vi "Run.vi"(0 "reg in":refnum<class "bronkhorst_reg_2.lvclass">, 1 "XB24 (F)":bool, 5 "ZY_control":T5={"Start"=FALSE, "Z_HSw"=0, "Z_HSetState"=enum."on", "Y_HSw"=0, "Y_HSetState"=enum."hand", "SP"=0.0, "Y_H"=0.0, "Reset_ALR"=FALSE} {"Y_H" step=1.0; "SP" step=0.01 format="%.2f"}, 7 "Y_in":dbl step=0.01 format="%.2f", 9 "Y_State":T4) -> (4 "reg out":refnum<class "bronkhorst_reg_2.lvclass">, 6 "Y":T1={"Y_Source"=enum."hand", "Y_SetState"=enum."hand", "SP_Set"=0.0, "SP"=0.0, "PV"=0.0, "PV_State"={"code"=0, "visible"=FALSE, "color"=0}, "Y_preSet"=0.0, "Y_Set"=0.0, "Y"=0.0, "Y_State"={"code"=0, "visible"=FALSE, "color"=0}, "YB"=FALSE} {"Y" format="%.2f"; "Y_preSet" format="%.2f"; "SP" step=0.01 format="%.2f"; "Y_Set" format="%.2f"; "PV" step=0.01 format="%.2f"; "SP_Set" step=0.01 format="%.2f"}, 8 "Y_out":dbl format="%.2f")   [LabVIEW 2019, in "control.lvlib" / "bronkhorst_reg_2.lvclass"]
uses:
  bronkhorst_reg_2.lvclass
  Inputs/Ctl/Parameter State short.ctl
  ctl/Y_Lim_State.ctl
  D:/my_projects/projects/Algorithms/Labview/19/Reg/Y_Limiter/Y_Limiter.lvclass
  ctl/ZY_control_short.ctl
  ctl/Z_State.ctl
  ctl/Y_state.ctl
  ctl/Y.ctl
  ctl/Y_source.ctl
  Y_Limiter/Y_Limiter.lvclass/Y_Limiter.ctl
  bronkhorst_reg_2.lvclass/bronkhorst_reg_2.ctl
  ctl/Y_control.ctl
  Inputs/Ctl/Sensor state.ctl
  Inputs/Ctl/Sensor alarm.ctl
  PID/PID Output Rate Limiter/PID Output Rate Limiter.lvclass/PID Output Rate Limiter.ctl
  PID/PID Timing Estimation/PID Timing Estimation.lvclass/PID Timing Estimation.ctl
  PID/PID Output Rate Limiter/PID Output Rate Limiter.vi
  PID/PID Output Rate Limiter/Read output.vi
  PID/PID Output Rate Limiter/Write output rate.vi
  PID/PID Output Rate Limiter/Read output rate.vi
  PID/PID Timing Estimation/PID Timing Estimation.vi
  Y_Limiter/Y_Limiter.lvclass
  D:/my_projects/projects/Algorithms/Labview/19/Reg/PID/PID Output Rate Limiter/PID Output Rate Limiter.lvclass
  PID/PID Output Rate Limiter/PID Output Rate Limiter.lvclass
  D:/my_projects/projects/Algorithms/Labview/19/Reg/PID/PID Timing Estimation/PID Timing Estimation.lvclass
  control.lvlib
  Inputs/Inputs.lvlib
panel:
  out "YLim_State":T7=enum."increase"
  out "End":bool
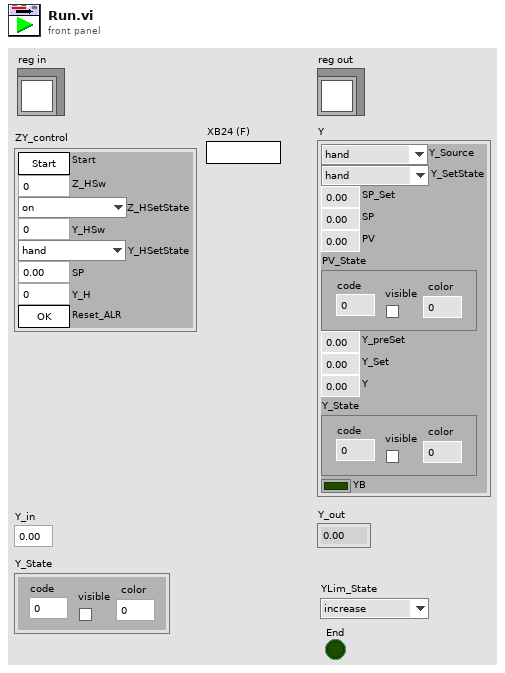
[diagram p1: front panel]
types:
  T1 = typedef "control.lvlib/Y.ctl" = cluster{"Y_Source":T2, "Y_SetState":T3, "SP_Set":dbl, "SP":dbl, "PV":dbl, "PV_State":T4, "Y_preSet":dbl, "Y_Set":dbl, "Y":dbl, "Y_State":T4, "YB":bool}
  T2 = typedef "control.lvlib/Y_source.ctl" = enum8{"initialize", "local disabled", "local hand", "hand", "auto", "dist"}
  T3 = typedef "control.lvlib/Y_state.ctl" = enum8{"initialize", "alarm", "min", "stop", "hand", "auto", "max"}
  T4 = typedef "Inputs.lvlib/Parameter State short.ctl" = cluster{"code":i32, "visible":bool, "color":u32}
  T5 = typedef "control.lvlib/ZY_control_short.ctl" = cluster{"Start":bool, "Z_HSw":u32, "Z_HSetState":T6, "Y_HSw":u32, "Y_HSetState":T3, "SP":dbl, "Y_H":dbl, "Reset_ALR":bool}
  T6 = typedef "control.lvlib/Z_State.ctl" = enum8{"initialization", "alarm", "disabled", "not ready", "stop ready", "reserv", "switched off", "reserv2", "switched on", "check", "on min", "decrease out", "on", "increase out", "on max"}
  T7 = typedef "control.lvlib/Y_Lim_State.ctl" = enum8{"initialization", "alarm", "stop", "decrease", "increase"}
  T8 = typedef "control.lvlib/Y_control.ctl" = cluster{"Y_HSw":u32, "Y_HSetState":T3, "Y_ASetState":T3, "Y_DSetState":T3}
  T9 = typedef "Inputs.lvlib/Sensor state.ctl" = cluster{"source":string, "color":u32, "visible":bool}[]
  T10 = typedef "Inputs.lvlib/Sensor alarm.ctl" = cluster{"source":string, "color":u32, "visible":bool}[]
  T11 = enum8{"alarm", "min", "stop", "hand", "auto", "max"}
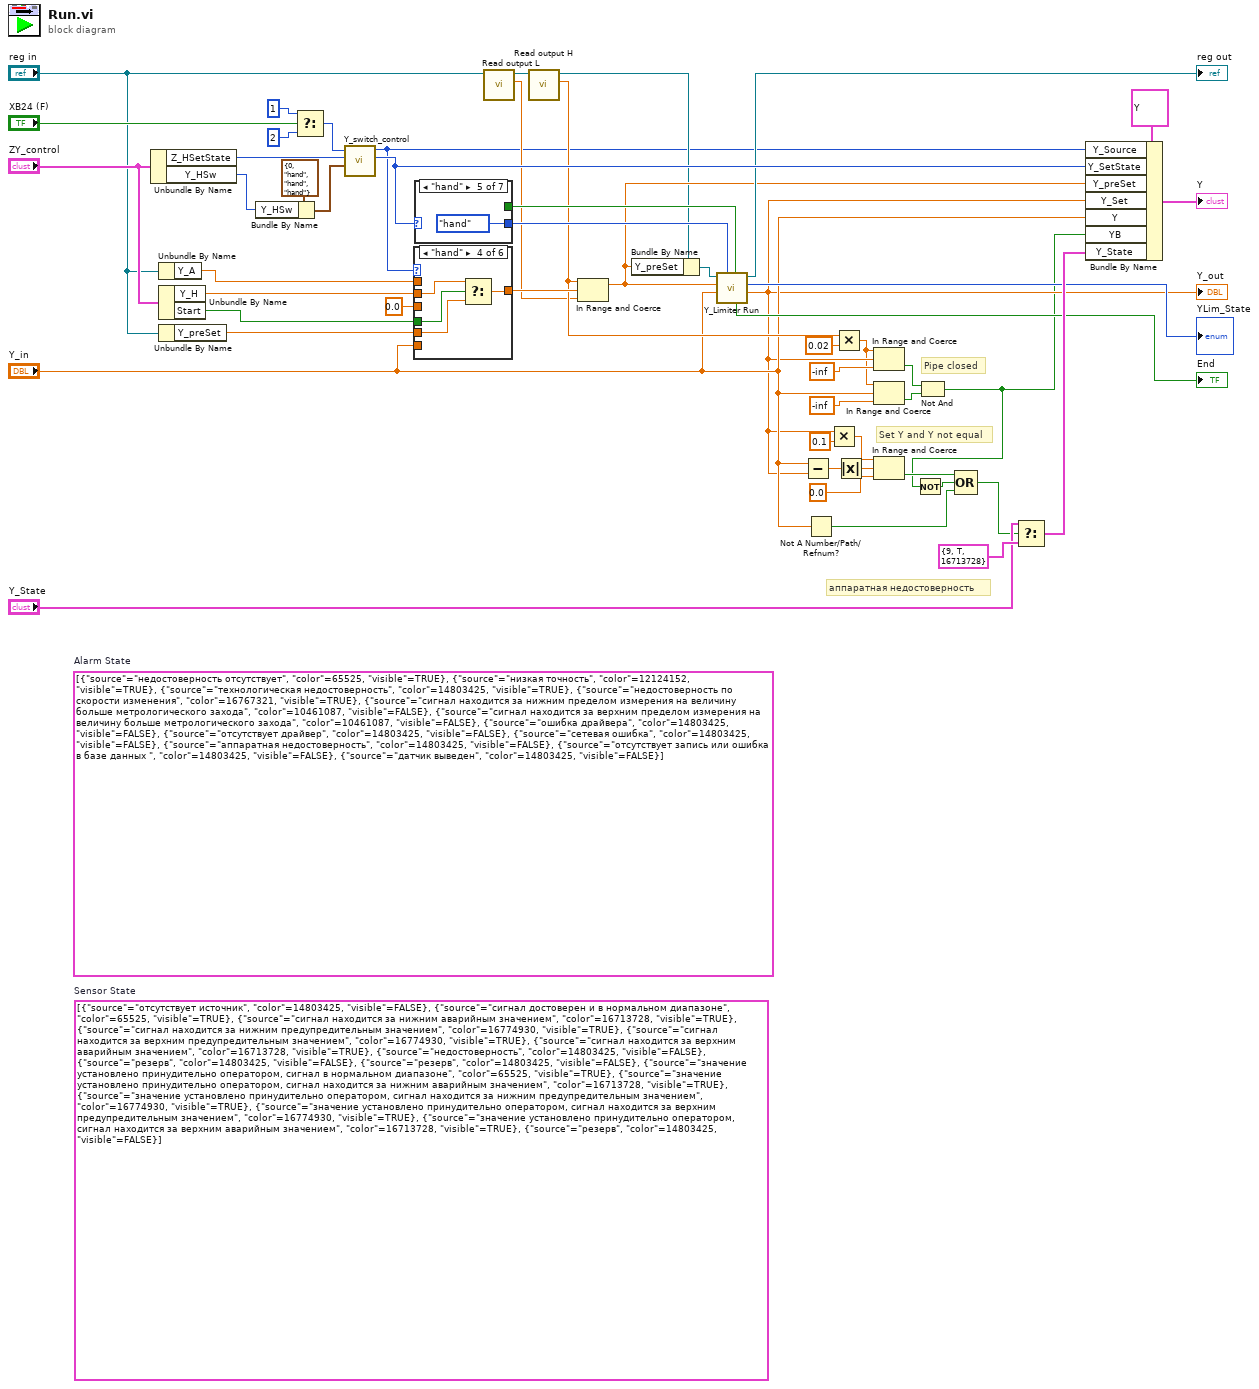
[diagram p0: block diagram]
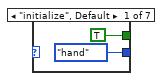
[diagram p2: hidden frame]
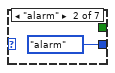
[diagram p3: hidden frame]
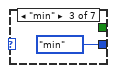
[diagram p4: hidden frame]
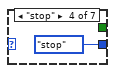
[diagram p5: hidden frame]
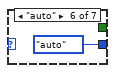
[diagram p6: hidden frame]
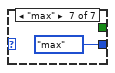
[diagram p7: hidden frame]
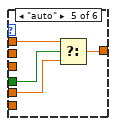
[diagram p11: hidden frame]
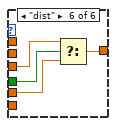
[diagram p12: hidden frame]
diagram:
  (unwired) T9 [{"source"="отсутствует источник", "color"=14803425, "visible"=FALSE}, {"source"="сигнал достоверен и в нормальном диапазоне", "color"=65525, "visible"=TRUE}, {"source"="сигнал находится за нижним аварийным значением", "color"=16713728, "visible"=TRUE}, {"source"="сигнал находится за нижним предупредительным значением", "color"=16774930, "visible"=TRUE}, {"source"="сигнал находится за верхним предупредительным значением", "color"=16774930, "visible"=TRUE}, {"source"="сигнал находится за верхним аварийным значением", "color"=16713728, "visible"=TRUE}, {"source"="недостоверность", "color"=14803425, "visible"=FALSE}, {"source"="резерв", "color"=14803425, "visible"=FALSE}, {"source"="резерв", "color"=14803425, "visible"=FALSE}, {"source"="значение установлено принудительно оператором, сигнал в нормальном диапазоне", "color"=65525, "visible"=TRUE}, {"source"="значение установлено принудительно оператором, сигнал находится за нижним аварийным значением", "color"=16713728, "visible"=TRUE}, {"source"="значение установлено принудительно оператором, сигнал находится за нижним предупредительным значением", "color"=16774930, "visible"=TRUE}, {"source"="значение установлено принудительно оператором, сигнал находится за верхним предупредительным значением", "color"=16774930, "visible"=TRUE}, {"source"="значение установлено принудительно оператором, сигнал находится за верхним аварийным значением", "color"=16713728, "visible"=TRUE}, {"source"="резерв", "color"=14803425, "visible"=FALSE}]  # Sensor State
  (unwired) T10 [{"source"="недостоверность отсутствует", "color"=65525, "visible"=TRUE}, {"source"="низкая точность", "color"=12124152, "visible"=TRUE}, {"source"="технологическая недостоверность", "color"=14803425, "visible"=TRUE}, {"source"="недостоверность по скорости изменения", "color"=16767321, "visible"=TRUE}, {"source"="сигнал находится за нижним пределом измерения на величину больше метрологического захода", "color"=10461087, "visible"=FALSE}, {"source"="сигнал находится за верхним пределом измерения на величину больше метрологического захода", "color"=10461087, "visible"=FALSE}, {"source"="ошибка драйвера", "color"=14803425, "visible"=FALSE}, {"source"="отсутствует драйвер", "color"=14803425, "visible"=FALSE}, {"source"="сетевая ошибка", "color"=14803425, "visible"=FALSE}, {"source"="аппаратная недостоверность", "color"=14803425, "visible"=FALSE}, {"source"="отсутствует запись или ошибка в базе данных ", "color"=14803425, "visible"=FALSE}, {"source"="датчик выведен", "color"=14803425, "visible"=FALSE}]  # Alarm State
  # "аппаратная недостоверность"
  # "Set Y and Y not equal"
  # "Pipe closed"
  n1 = Unbundle By Name("ZY_control") -> ("Z_HSetState"=w46:T6, "Y_HSw"=w47:u32)
  n2 = Unbundle By Name("reg in") -> ("Y_A"=w20:dbl)
  n3 = Unbundle By Name("ZY_control") -> ("Y_H"=w42:dbl, "Start"=w43:bool)
  n4 = Unbundle By Name("reg in") -> ("Y_preSet"=w21:dbl)
  n5 = Bundle By Name(cluster=T8 {"Y_HSw"=0, "Y_HSetState"=enum."hand", "Y_ASetState"=enum."hand", "Y_DSetState"=enum."hand"} ("Y"), "Y_HSw"=w47) -> (w45:T8)
  n6 = Select(t=u32 1, s="XB24 (F)", f=u32 2 ("Y_HSw")) -> (s? t:f=w50:u32)
  n7 = call "Y_switch_control.vi"("Y"=w45, "Z_State"=w46, "Y_LSw (2-auto)"=w50) -> ("Y_SetState"=w48:T3, "Y_Source"=w12:T2)  [unwired: 7 in]
  n8 = case shown="\"hand\"" w12 {
    tunnel: w42 -> [_ _ _ w56 _ _]
    tunnel: "Y_in" -> [w53 w54 w55 _ _ _]
    tunnel: 0.0 ("Y_A") -> [_ _ _ _ _ w66]
    tunnel: [w53 w54 w55 w59 w63 w67] -> w22
    tunnel: w20 -> [_ _ _ _ w60 _]
    tunnel: w21 -> [_ _ _ w58 w62 w65]
    tunnel: w43 -> [_ _ _ w57 w61 w64]
    frame "initialize", Default {
    }
    frame "local disabled" {
    }
    frame "local hand" {
    }
    frame "hand" {
      n9 = Select(t=w56, s=w57, f=w58) -> (s? t:f=w59:dbl)
    }
    frame "auto" {
      n10 = Select(t=w60, s=w61, f=w62) -> (s? t:f=w63:dbl)
    }
    frame "dist" {
      n11 = Select(t=w66, s=w64, f=w65) -> (s? t:f=w67:dbl)
    }
  }
  n12 = case shown="\"hand\"" w48 {
    tunnel: [T11."hand" ("X1(SetState)") T11."alarm" ("X1(SetState)") T11."min" ("X1(SetState)") T11."stop" ("X1(SetState)") T11."hand" ("X1(SetState)") T11."auto" ("X1(SetState)") T11."max" ("X1(SetState)")] -> w29
    tunnel: [TRUE _ _ _ _ _ _] -> w28
    frame "initialize", Default {
    }
    frame "alarm" {
    }
    frame "min" {
    }
    frame "stop" {
    }
    frame "hand" {
    }
    frame "auto" {
    }
    frame "max" {
    }
  }
  n13 = call "Read output L.vi"("Y_Limiter in"="reg in") -> ("output L"=w14:dbl, "Y_Limiter out"=w13:refnum<class "bronkhorst_reg_2.lvclass">)  [unwired: 9 in]
  n14 = call "Read output H.vi"("Y_Limiter in"=w13) -> ("output H"=w17:dbl, "Y_Limiter out"=w16:refnum<class "bronkhorst_reg_2.lvclass">)  [unwired: 9 in]
  n15 = In Range and Coerce(upper limit=w17, x=w22, lower limit=w14) -> (coerced(x)=w19:dbl)  [unwired: 1 out]
  n16 = Bundle By Name(cluster=w16, "Y_preSet"=w19) -> (w18:refnum<class "bronkhorst_reg_2.lvclass">)
  n17 = call "Y_Limiter Run.vi"("reinitialize? (F)"=w28, "X1(SetState)"=w29, "Y (NaN)"="Y_in", "Y_Set"=w19, "Y_Limiter in"=w18) -> ("output"=w6:dbl, "Y_Lim_State"=→"YLim_State":T7, "Y_Limiter out"=→"reg out":refnum<class "bronkhorst_reg_2.lvclass">, "End"=→"End":bool)  [unwired: 3 in]
  "Y_out" <- w6
  n18 = Subtract(x="Y_in", y=w6) -> (x-y=w36:dbl)
  n19 = Not A Number/Path/Refnum?(number/path/refnum="Y_in") -> (NaN/Path/Refnum?=w3:bool)
  n20 = Multiply(x=w6, y=0.1) -> (x*y=w10:dbl)
  n21 = Multiply(x=w17, y=0.02) -> (x*y=w5:dbl)
  n22 = Absolute Value(x=w36) -> (abs(x)=w9:dbl)
  n23 = In Range and Coerce(upper limit=w5, x=w6, lower limit=-inf) -> (In Range?=w38:bool)  [unwired: 1 out]
  n24 = In Range and Coerce(upper limit=w5, x="Y_in", lower limit=-inf) -> (In Range?=w37:bool)  [unwired: 1 out]
  n25 = In Range and Coerce(upper limit=w10, x=w9, lower limit=0.0) -> (In Range?=w4:bool)  [unwired: 1 out]
  n26 = Not And(1:w37, 2:w38) -> (0:w1:bool)
  n27 = Not(x=w1) -> (.not. x?=w2:bool)
  n28 = Compound Arithmetic op=OR(w4, w2, w3) -> (w33:bool)
  n29 = Select(t="Y_State", s=w33, f=cluster{"code":i32, "visible":bool, "color":u32} {"code"=9, "visible"=TRUE, "color"=16713728}) -> (s? t:f=w32:T4)
  n30 = Bundle By Name(cluster=T1 {"Y_Source"=enum."initialize", "Y_SetState"=enum."initialize", "SP_Set"=0.0, "SP"=0.0, "PV"=0.0, "PV_State"={"code"=0, "visible"=FALSE, "color"=0}, "Y_preSet"=0.0, "Y_Set"=0.0, "Y"=0.0, "Y_State"={"code"=0, "visible"=FALSE, "color"=0}, "YB"=FALSE} ("Y_State"), "Y_Source"=w12, "Y_SetState"=w48, "Y_preSet"=w19, "Y_Set"=w6, "Y"="Y_in", "YB"=w1, "Y_State"=w32) -> (→"Y":T1)
